vi "Calc_ISO_WeekNumber.vi"(8 "error in (no error)":errorcluster, 11 "Date (now)":timestamp) -> (0 "error out":errorcluster, 1 "ISO week number":i32, 2 "SBZ year 2 digits":i32, 3 "SBZ year 4 digits":i32, 4 "Real year 4 digits":i32, 5 "Date ISO":T1, 6 "Real year 2 digits":i32)   [LabVIEW 2018]
doc: "Ce VI calcule le n° de semaine selon la norme ISO 8601.\nEn plus, il donne en sortie l'année, soit en 2, soit en 4 digits.\nL'année est enfin donnée en 2 versions:\n- l'année réelle (qui change au 1er janvier!)\n- l'année \"SBZ\" qui change avec le n° de semaine (sem. 1).\n\n\n<B>Date (now)</B> : horodatage. Actuel si non défini.\n\n\n<B>Date ISO</B> : date complète (cluster LabVIEW)\n\n<B>Année SBZ 4 digits</B> : année changeant avec le n° de semaine 1, format du type \"2006\".\n\n<B>Année SBZ 2 digits</B> : année changeant avec le n° de semaine 1, format du type \"06\".\n\n<B>N° semaine ISO</B> : numéro de semaine dans l'année, selon ISO 8601\n\n<B>Année réelle 4 digits</B> : année changeant le 1er janvier, format du type \"2006\".\n\n<B>Année réelle 2 digits</B> : année changeant le 1er janvier, format du type \"06\".\n\n\nJ. Bögli / P.-A. Glardon Sonceboz SA\nJanvier 2006\nAdaptation d'un VI de Rolf Kalbermatter"
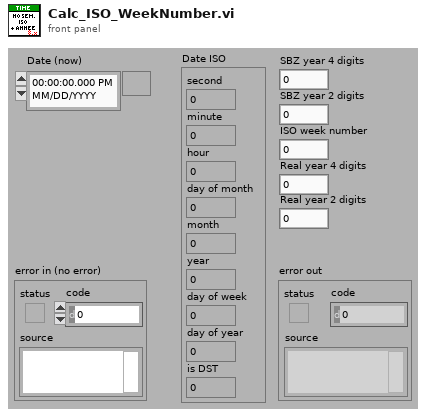
[diagram p1: front panel]
types:
  T1 = cluster{"second":i32, "minute":i32, "hour":i32, "day of month":i32, "month":i32, "year":i32, "day of week":i32, "day of year":i32, "is DST":i32}
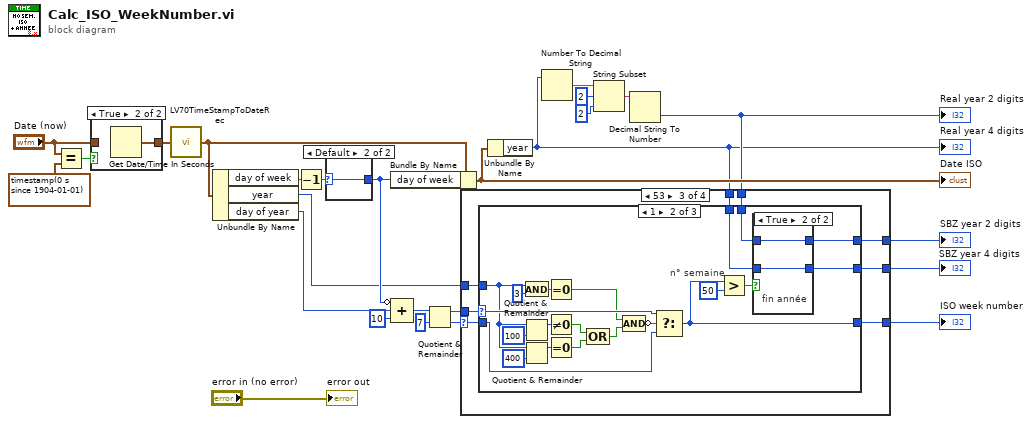
[diagram p0: block diagram]
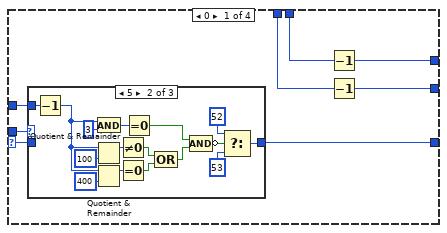
[diagram p2: hidden frame]
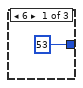
[diagram p3: hidden frame]
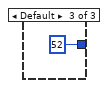
[diagram p4: hidden frame]
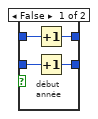
[diagram p7: hidden frame]
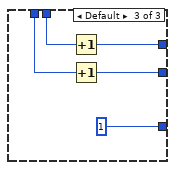
[diagram p8: hidden frame]
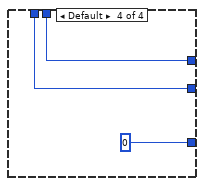
[diagram p9: hidden frame]
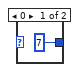
[diagram p10: hidden frame]
diagram:
  n1 = Equal?(x="Date (now)", y=timestamp(0 s since 1904-01-01) ("seconds (now)")) -> (x = y?=w24:bool)
  n2 = case shown="True" w24 {
    tunnel: [w27 w28] -> w25
    tunnel: "Date (now)" -> [w27 _]
    frame False {
    }
    frame True {
      n3 = Get Date/Time In Seconds() -> (seconds since 1Jan1904=w28:timestamp)
    }
  }
  n4 = call <vilib>:"LV70TimeStampToDateRec.vi"("time stamp"=w25) -> ("date time rec"=w26:T1)
  n5 = Unbundle By Name(w26) -> ("day of week"=w19:i32, "year"=w14:i32, "day of year"=w13:i32)
  n6 = Decrement(x=w19) -> (x-1=w20:i32)
  n7 = case shown="Default" w20 {
    selector: w20 -> [_ w30]
    tunnel: [7 ("day of week") w30] -> w18
    frame 0 {
    }
    frame Default {
    }
  }
  n8 = Bundle By Name(cluster=w26, "day of week"=w18) -> (w12:T1)
  "Date ISO" <- w12
  n9 = Compound Arithmetic op=ADD(invert w18, w13, 10 ("Input")) -> (w22:i32)
  n10 = Quotient & Remainder(x=w22, y=7) -> (x-y*floor(x/y)=w16:i32, floor(x/y)=w17:i32)
  n11 = Unbundle By Name(w12) -> ("year"=w3:i32)
  "Real year 4 digits" <- w3
  n12 = Number To Decimal String(number=w3) -> (decimal integer string=w9:string)  [unwired: 1 in]
  n13 = String Subset(string=w9, offset (0)=2, length (rest)=2 ("length (rest)")) -> (substring=w8:string)
  n14 = Decimal String To Number(string=w8) -> (number=w4:i32)  [unwired: 2 in, 1 out]
  "Real year 2 digits" <- w4
  n15 = case shown="53" w17 {
    selector: w17 -> [w38 w59 w65 _]
    tunnel: [w36 w59 w66 0] -> w15
    tunnel: w16 -> [w37 _ w67 _]
    tunnel: w14 -> [w35 _ w64 _]
    tunnel: w4 -> [w33 w58 w63 w104]
    tunnel: w3 -> [w31 w57 w62 w103]
    tunnel: [w34 w58 w61 w104] -> w2
    tunnel: [w32 w57 w60 w103] -> w1
    frame 0 {
      n16 = case shown="5" w37 {
        tunnel: [53 w55 52 ("t")] -> w36
        tunnel: w38 -> [_ _ _]
        tunnel: w35 -> [_ w43 _]
        frame 6 {
        }
        frame 5 {
          n17 = Decrement(x=w43) -> (x-1=w42:i32)
          n18 = And(x=w42, y=3) -> (x .and. y?=w51:i32)
          n19 = Quotient & Remainder(x=w42, y=100) -> (x-y*floor(x/y)=w52:i32)  [unwired: 1 out]
          n20 = Quotient & Remainder(x=w42, y=400) -> (x-y*floor(x/y)=w53:i32)  [unwired: 1 out]
          n21 = Not Equal To 0?(x=w52) -> (x != 0?=w40:bool)
          n22 = Equal To 0?(x=w53) -> (x = 0?=w41:bool)
          n23 = Equal To 0?(x=w51) -> (x = 0?=w54:bool)
          n24 = Compound Arithmetic op=OR(w40, w41) -> (w47:bool)
          n25 = Compound Arithmetic op=AND(w54, w47) -> (invert w48:bool)
          n26 = Select(t=52, s=w48, f=53 ("t")) -> (s? t:f=w55:i32)
        }
        frame Default {
        }
      }
      n27 = Decrement(x=w33) -> (x-1=w34:i32)
      n28 = Decrement(x=w31) -> (x-1=w32:i32)
    }
    frame 1..52 {
    }
    frame 53 {
      n29 = case shown="1" w67 {
        selector: w67 -> [_ w91 _]
        tunnel: [w70 w72 1] -> w66
        tunnel: w65 -> [w70 w90 _]
        tunnel: w64 -> [_ w78 _]
        tunnel: w63 -> [w69 w76 w101]
        tunnel: w62 -> [w68 w74 w100]
        tunnel: [w69 w77 w99] -> w61
        tunnel: [w68 w75 w98] -> w60
        frame 0 {
        }
        frame 1 {
          # "n° semaine"
          n30 = And(x=w78, y=3) -> (x .and. y?=w86:i32)
          n31 = Quotient & Remainder(x=w78, y=100) -> (x-y*floor(x/y)=w87:i32)  [unwired: 1 out]
          n32 = Quotient & Remainder(x=w78, y=400) -> (x-y*floor(x/y)=w88:i32)  [unwired: 1 out]
          n33 = Equal To 0?(x=w86) -> (x = 0?=w89:bool)
          n34 = Not Equal To 0?(x=w87) -> (x != 0?=w81:bool)
          n35 = Equal To 0?(x=w88) -> (x = 0?=w80:bool)
          n36 = Compound Arithmetic op=OR(w81, w80) -> (w79:bool)
          n37 = Compound Arithmetic op=AND(w89, w79) -> (invert w82:bool)
          n38 = Select(t=w91, s=w82, f=w90) -> (s? t:f=w72:i32)
          n39 = Greater?(x=w72, y=50) -> (0:w73:bool)
          n40 = case shown="True" w73 {
            tunnel: [w95 w97] -> w77
            tunnel: w76 -> [w94 w97]
            tunnel: [w93 w96] -> w75
            tunnel: w74 -> [w92 w96]
            frame False {
              # "début\nannée"
              n41 = Increment(x=w94) -> (x+1=w95:i32)
              n42 = Increment(x=w92) -> (x+1=w93:i32)
            }
            frame True {
              # "fin année"
            }
          }
        }
        frame Default {
          n43 = Increment(x=w101) -> (x+1=w99:i32)
          n44 = Increment(x=w100) -> (x+1=w98:i32)
        }
      }
    }
    frame Default {
    }
  }
  "ISO week number" <- w15
  "SBZ year 4 digits" <- w1
  "SBZ year 2 digits" <- w2
  "error out" <- "error in (no error)"
